vi "Actualizar ListBox.vi"(8 "error in (no error)":errorcluster, 9 "Tabla":string[][](table) caption="Result Set (from first statement with results)", 10 "Multicolumn Listbox 2":refnum<vi>, 11 "Turnos in":refnum<class "Turnos.lvclass">) -> (0 "error out":errorcluster, 3 "Turnos out":refnum<class "Turnos.lvclass">)   [LabVIEW 2020, in "Turnos.lvlib" / "Turnos.lvclass"]
uses:
  Turnos.lvclass
  Turnos.lvclass/Turnos.ctl
panel:
  out "String":string
  in  "array w/ subset deleted":string[][](array[string])
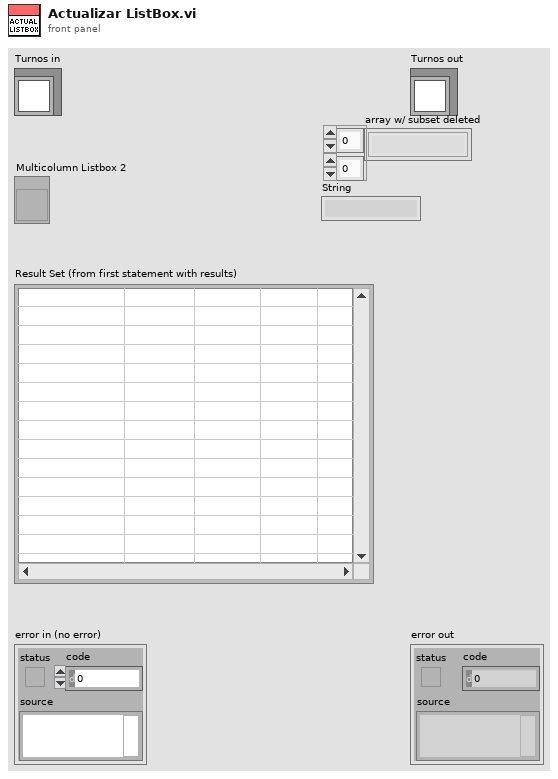
[diagram p1: front panel]
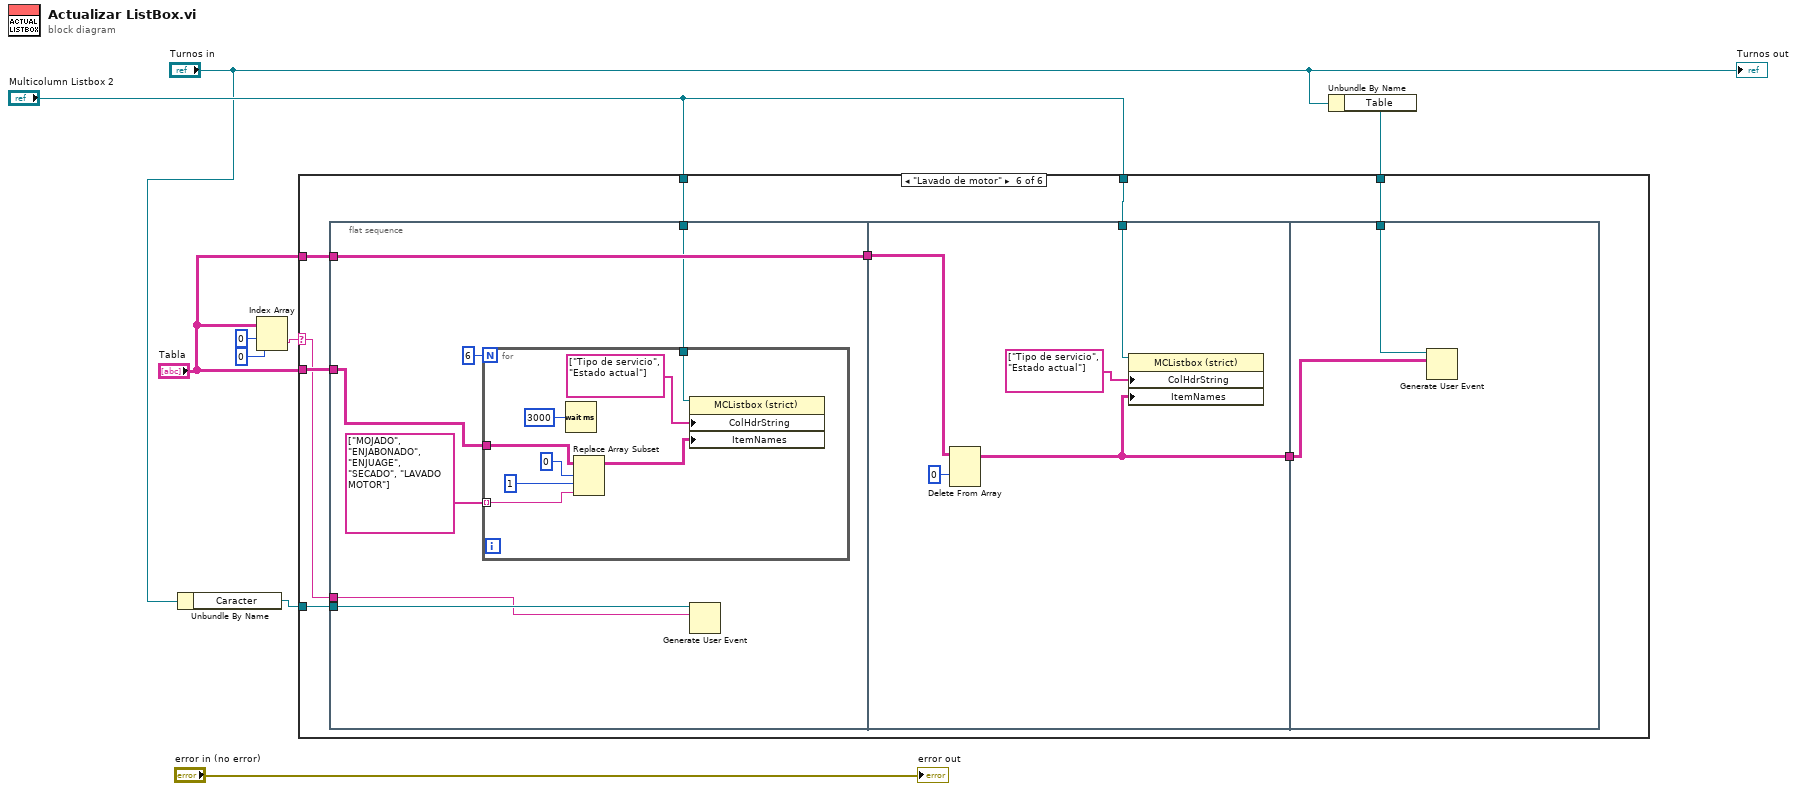
[diagram p0: block diagram]
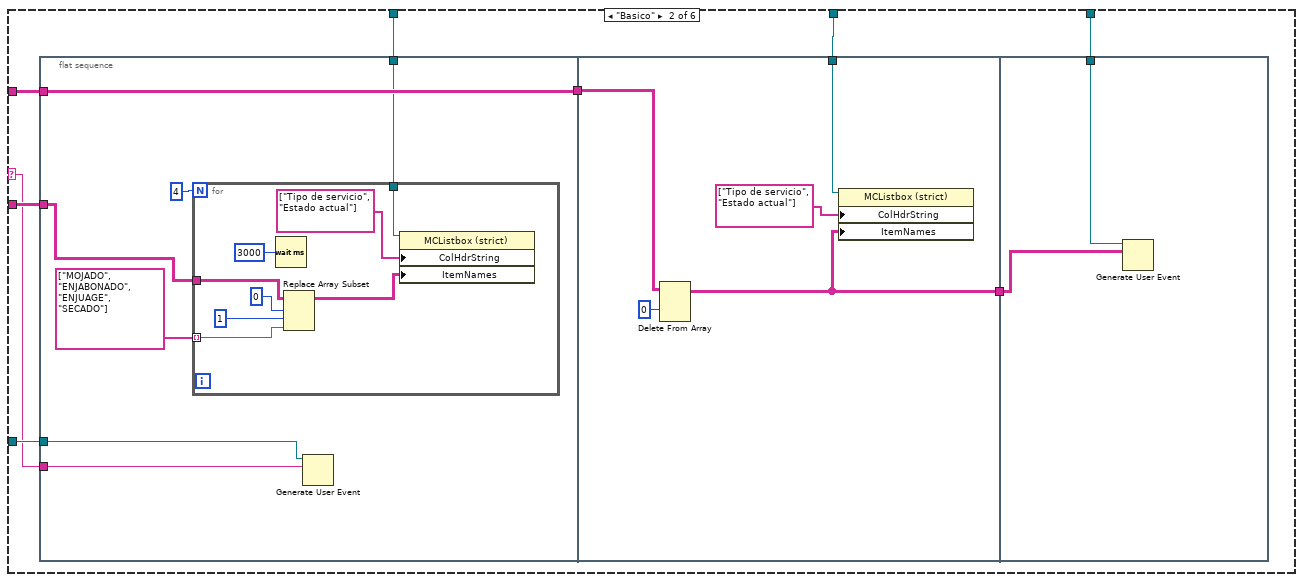
[diagram p3: hidden frame]
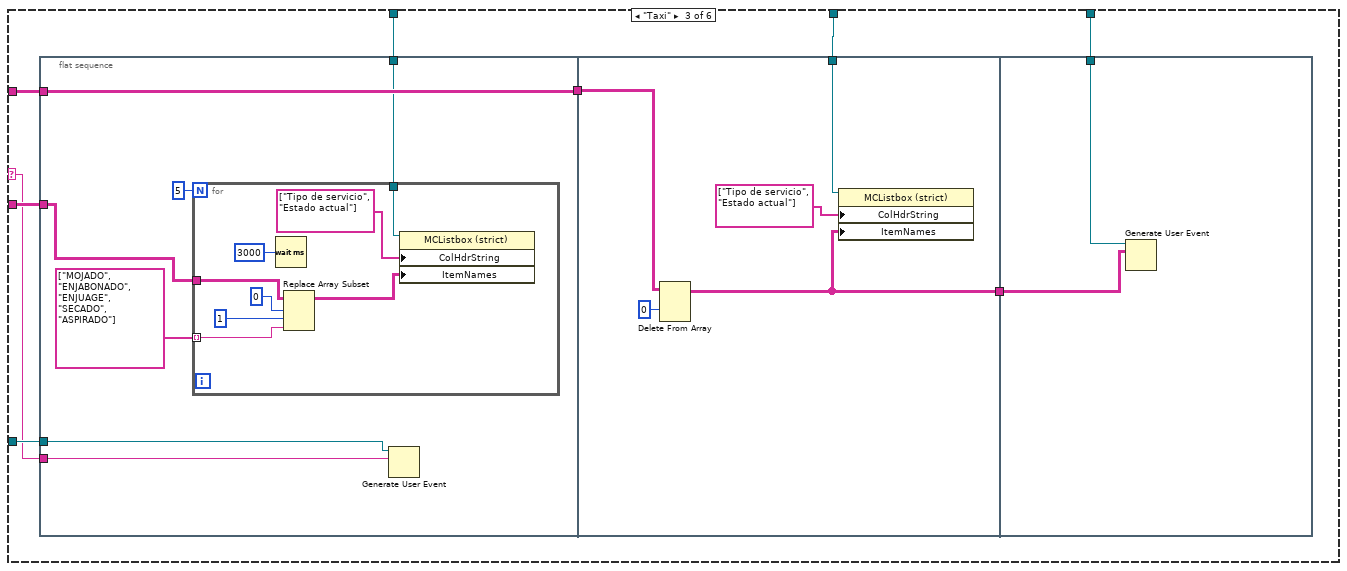
[diagram p4: hidden frame]
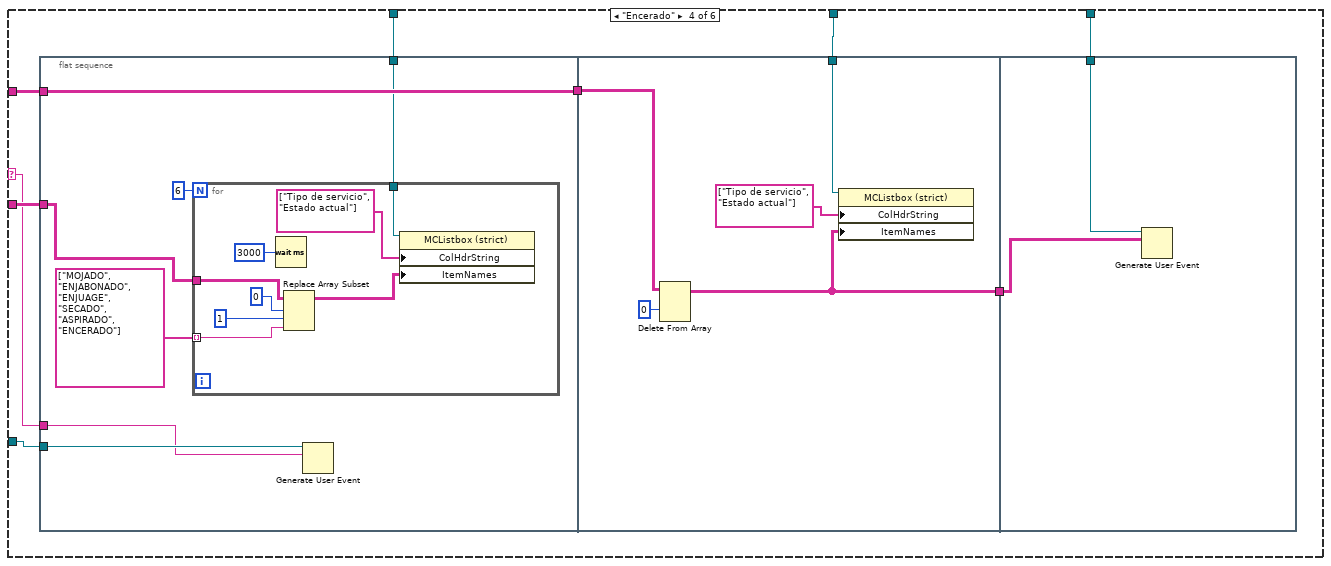
[diagram p5: hidden frame]
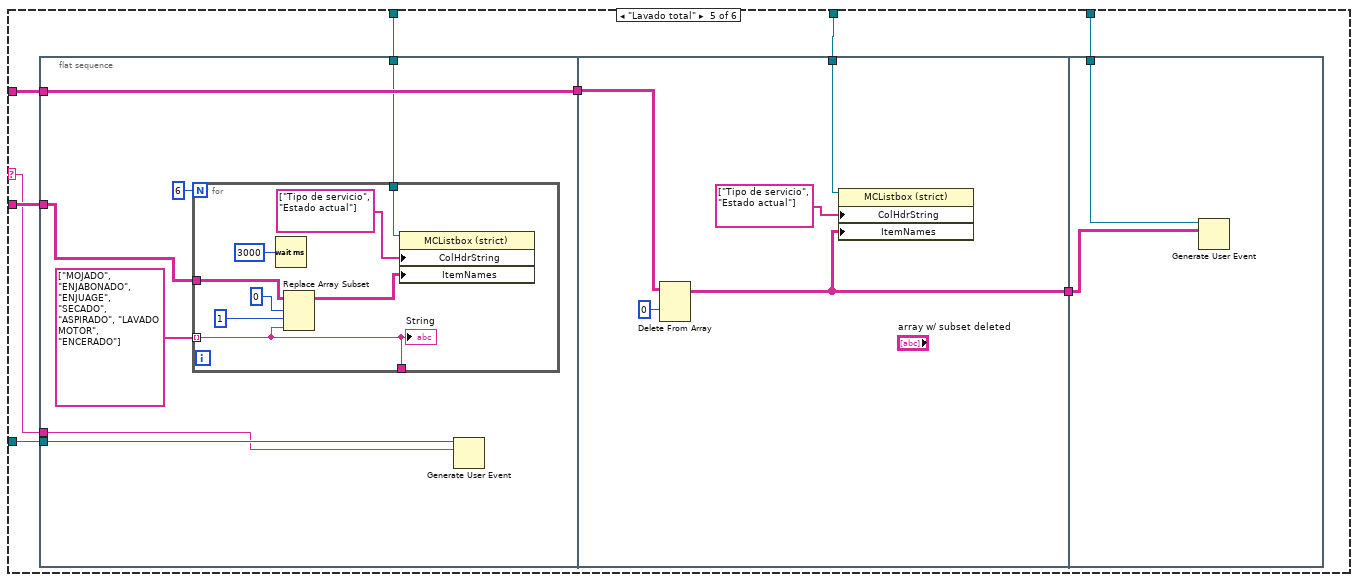
[diagram p6: hidden frame]
diagram:
  n1 = Unbundle By Name("Turnos in") -> ("Caracter"=w1:refnum<user-event>)
  n2 = Index Array(array="Tabla", index (row)=0 ("index"), index (col)=0 ("disabled index (col)")) -> (element=w3:string)
  n3 = Unbundle By Name("Turnos in") -> ("Table"=w7:refnum<user-event>)
  n4 = case shown="\"Lavado de motor\"" w3 {
    selector: w3 -> [_ w10 w41 w72 w103 w134]
    tunnel: "Tabla" -> [_ w18 w49 w80 w111 w142]
    tunnel: "Tabla" -> [_ w17 w48 w79 w110 w141]
    tunnel: "Multicolumn Listbox 2" -> [_ w15 w46 w77 w108 w139]
    tunnel: "Multicolumn Listbox 2" -> [_ w14 w45 w76 w107 w138]
    tunnel: w7 -> [_ w12 w43 w74 w105 w136]
    tunnel: w1 -> [_ w11 w42 w73 w104 w135]
    frame "False", Default {
    }
    frame "Basico" {
      n5 = flat-sequence {
        tunnel: w18 -> [w23]
        tunnel: w17 -> [w22]
        tunnel: [w22] -> w16
        tunnel: w14 -> [w21]
        tunnel: w11 -> [w20]
        tunnel: w10 -> [w19]
        tunnel: w16 -> [w36]
        tunnel: w15 -> [w38]
        tunnel: [w34] -> w13
        tunnel: w13 -> [w40]
        tunnel: w12 -> [w39]
        frame #0 {
          n6 = for {
            N: 4 -> [_]
            tunnel: w23 -> [w33]
            tunnel: string[] ["MOJADO", "ENJABONADO", "ENJUAGE", "SECADO"] -> [w26] mode=indexing
            tunnel: w21 -> [w27]
            n7 = Wait (ms)(milliseconds to wait=u32 3000) -> ()  [unwired: 1 out]
            n8 = Replace Array Subset(array=w33, new element=w26, index (row)=0, index (col)=1 ("disabled index (col)")) -> (w28:string[][])
            n9 = property on="Property Node" class="MCListbox (strict)"(reference=w27, "ColHdrString"=string[] ["Tipo de servicio", "Estado actual"] ("Column Header Strings[]"), "ItemNames"=w28) -> ()  [unwired: 1 in, 2 out]
          }
          n10 = Generate User Event(user event=w20, event data cluster=w19) -> ()  [unwired: 2 in, 2 out]
        }
        frame #1 {
          n11 = Delete From Array(array=w36, index (row)=0) -> (array with subset deleted=w34:string[][])  [unwired: 2 in, 1 out]
          n12 = property on="Property Node" class="MCListbox (strict)"(reference=w38, "ColHdrString"=string[] ["Tipo de servicio", "Estado actual"] ("Column Header Strings[]"), "ItemNames"=w34) -> ()  [unwired: 1 in, 2 out]
        }
        frame #2 {
          n13 = Generate User Event(user event=w39, event data cluster=w40) -> ()  [unwired: 2 in, 2 out]
        }
      }
    }
    frame "Taxi" {
      n14 = flat-sequence {
        tunnel: w49 -> [w54]
        tunnel: w48 -> [w53]
        tunnel: [w53] -> w47
        tunnel: w45 -> [w52]
        tunnel: w42 -> [w51]
        tunnel: w41 -> [w50]
        tunnel: w47 -> [w67]
        tunnel: w46 -> [w69]
        tunnel: [w65] -> w44
        tunnel: w44 -> [w70]
        tunnel: w43 -> [w71]
        frame #0 {
          n15 = for {
            N: 5 -> [_]
            tunnel: w54 -> [w64]
            tunnel: string[] ["MOJADO", "ENJABONADO", "ENJUAGE", "SECADO", "ASPIRADO"] -> [w57] mode=indexing
            tunnel: w52 -> [w58]
            n16 = Wait (ms)(milliseconds to wait=u32 3000) -> ()  [unwired: 1 out]
            n17 = Replace Array Subset(array=w64, new element=w57, index (row)=0, index (col)=1 ("disabled index (col)")) -> (w59:string[][])
            n18 = property on="Property Node" class="MCListbox (strict)"(reference=w58, "ColHdrString"=string[] ["Tipo de servicio", "Estado actual"] ("Column Header Strings[]"), "ItemNames"=w59) -> ()  [unwired: 1 in, 2 out]
          }
          n19 = Generate User Event(user event=w51, event data cluster=w50) -> ()  [unwired: 2 in, 2 out]
        }
        frame #1 {
          n20 = Delete From Array(array=w67, index (row)=0) -> (array with subset deleted=w65:string[][])  [unwired: 2 in, 1 out]
          n21 = property on="Property Node" class="MCListbox (strict)"(reference=w69, "ColHdrString"=string[] ["Tipo de servicio", "Estado actual"] ("Column Header Strings[]"), "ItemNames"=w65) -> ()  [unwired: 1 in, 2 out]
        }
        frame #2 {
          n22 = Generate User Event(user event=w71, event data cluster=w70) -> ()  [unwired: 2 in, 2 out]
        }
      }
    }
    frame "Encerado" {
      n23 = flat-sequence {
        tunnel: w80 -> [w85]
        tunnel: w79 -> [w84]
        tunnel: [w84] -> w78
        tunnel: w76 -> [w83]
        tunnel: w73 -> [w82]
        tunnel: w72 -> [w81]
        tunnel: w78 -> [w98]
        tunnel: w77 -> [w100]
        tunnel: [w96] -> w75
        tunnel: w75 -> [w102]
        tunnel: w74 -> [w101]
        frame #0 {
          n24 = for {
            N: 6 -> [_]
            tunnel: w85 -> [w95]
            tunnel: string[] ["MOJADO", "ENJABONADO", "ENJUAGE", "SECADO", "ASPIRADO", "ENCERADO"] -> [w88] mode=indexing
            tunnel: w83 -> [w89]
            n25 = Wait (ms)(milliseconds to wait=u32 3000) -> ()  [unwired: 1 out]
            n26 = Replace Array Subset(array=w95, new element=w88, index (row)=0, index (col)=1 ("disabled index (col)")) -> (w90:string[][])
            n27 = property on="Property Node" class="MCListbox (strict)"(reference=w89, "ColHdrString"=string[] ["Tipo de servicio", "Estado actual"] ("Column Header Strings[]"), "ItemNames"=w90) -> ()  [unwired: 1 in, 2 out]
          }
          n28 = Generate User Event(user event=w82, event data cluster=w81) -> ()  [unwired: 2 in, 2 out]
        }
        frame #1 {
          n29 = Delete From Array(array=w98, index (row)=0) -> (array with subset deleted=w96:string[][])  [unwired: 2 in, 1 out]
          n30 = property on="Property Node" class="MCListbox (strict)"(reference=w100, "ColHdrString"=string[] ["Tipo de servicio", "Estado actual"] ("Column Header Strings[]"), "ItemNames"=w96) -> ()  [unwired: 1 in, 2 out]
        }
        frame #2 {
          n31 = Generate User Event(user event=w101, event data cluster=w102) -> ()  [unwired: 2 in, 2 out]
        }
      }
    }
    frame "Lavado total" {
      n32 = flat-sequence {
        tunnel: w111 -> [w116]
        tunnel: w110 -> [w115]
        tunnel: [w115] -> w109
        tunnel: w107 -> [w114]
        tunnel: w104 -> [w113]
        tunnel: w103 -> [w112]
        tunnel: w109 -> [w129]
        tunnel: w108 -> [w131]
        tunnel: [w127] -> w106
        tunnel: w106 -> [w132]
        tunnel: w105 -> [w133]
        frame #0 {
          n33 = for {
            N: 6 -> [_]
            tunnel: w116 -> [w126]
            tunnel: string[] ["MOJADO", "ENJABONADO", "ENJUAGE", "SECADO", "ASPIRADO", "LAVADO MOTOR", "ENCERADO"] -> [w119] mode=indexing
            tunnel: w114 -> [w120]
            tunnel: [w119] -> _
            n34 = Wait (ms)(milliseconds to wait=u32 3000) -> ()  [unwired: 1 out]
            n35 = Replace Array Subset(array=w126, new element=w119, index (row)=0, index (col)=1 ("disabled index (col)")) -> (w121:string[][])
            n36 = property on="Property Node" class="MCListbox (strict)"(reference=w120, "ColHdrString"=string[] ["Tipo de servicio", "Estado actual"] ("Column Header Strings[]"), "ItemNames"=w121) -> ()  [unwired: 1 in, 2 out]
            "String" <- w119
          }
          n37 = Generate User Event(user event=w113, event data cluster=w112) -> ()  [unwired: 2 in, 2 out]
        }
        frame #1 {
          n38 = Delete From Array(array=w129, index (row)=0) -> (array with subset deleted=w127:string[][])  [unwired: 2 in, 1 out]
          n39 = property on="Property Node" class="MCListbox (strict)"(reference=w131, "ColHdrString"=string[] ["Tipo de servicio", "Estado actual"] ("Column Header Strings[]"), "ItemNames"=w127) -> ()  [unwired: 1 in, 2 out]
        }
        frame #2 {
          n40 = Generate User Event(user event=w133, event data cluster=w132) -> ()  [unwired: 2 in, 2 out]
        }
      }
    }
    frame "Lavado de motor" {
      n41 = flat-sequence {
        tunnel: w142 -> [w147]
        tunnel: w141 -> [w146]
        tunnel: [w146] -> w140
        tunnel: w138 -> [w145]
        tunnel: w135 -> [w144]
        tunnel: w134 -> [w143]
        tunnel: w140 -> [w160]
        tunnel: w139 -> [w162]
        tunnel: [w158] -> w137
        tunnel: w137 -> [w164]
        tunnel: w136 -> [w163]
        frame #0 {
          n42 = for {
            N: 6 -> [_]
            tunnel: w147 -> [w157]
            tunnel: string[] ["MOJADO", "ENJABONADO", "ENJUAGE", "SECADO", "LAVADO MOTOR"] -> [w150] mode=indexing
            tunnel: w145 -> [w151]
            n43 = Wait (ms)(milliseconds to wait=u32 3000) -> ()  [unwired: 1 out]
            n44 = Replace Array Subset(array=w157, new element=w150, index (row)=0, index (col)=1 ("disabled index (col)")) -> (w152:string[][])
            n45 = property on="Property Node" class="MCListbox (strict)"(reference=w151, "ColHdrString"=string[] ["Tipo de servicio", "Estado actual"] ("Column Header Strings[]"), "ItemNames"=w152) -> ()  [unwired: 1 in, 2 out]
          }
          n46 = Generate User Event(user event=w144, event data cluster=w143) -> ()  [unwired: 2 in, 2 out]
        }
        frame #1 {
          n47 = Delete From Array(array=w160, index (row)=0) -> (array with subset deleted=w158:string[][])  [unwired: 2 in, 1 out]
          n48 = property on="Property Node" class="MCListbox (strict)"(reference=w162, "ColHdrString"=string[] ["Tipo de servicio", "Estado actual"] ("Column Header Strings[]"), "ItemNames"=w158) -> ()  [unwired: 1 in, 2 out]
        }
        frame #2 {
          n49 = Generate User Event(user event=w163, event data cluster=w164) -> ()  [unwired: 2 in, 2 out]
        }
      }
    }
  }
  "error out" <- "error in (no error)"
  "Turnos out" <- "Turnos in"
